vi "LSX Set Command Timeout.vi"(7 "lAtoCalibrate":i32, 8 "error in (no error)":errorcluster, 9 "lAtoMove":i32, 10 "lAtoRead":i32, 11 "lLSID":i32) -> (0 "error out":errorcluster, 3 "function return":i32)   [LabVIEW 2018, in "Tango.lvlib"]
doc: "TANGOAPI int TANGOCALL LSX_SetCommandTimeout (int lLSID, int lAtoRead, int lAtoMove, int lAtoCalibrate);"
uses:
  Tango.lvlib
  SubVIs/Tango_DLL.dll
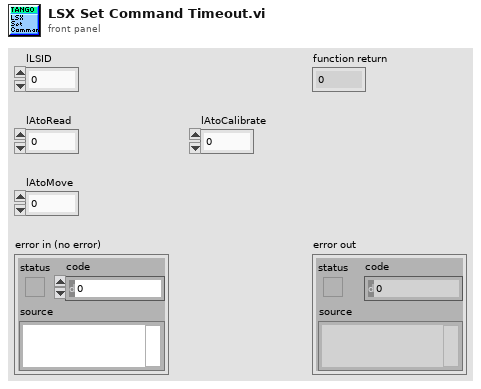
[diagram p1: front panel]
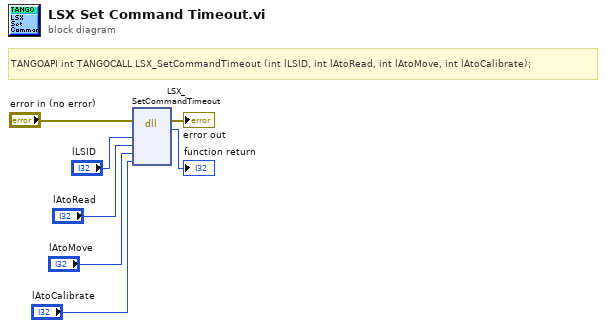
[diagram p0: block diagram]
diagram:
  # "TANGOAPI int TANGOCALL LSX_SetCommandTimeout (int lLSID, int lAtoRead, int lAtoMove, int lAtoCalibrate);"
  n1 = dll-call lib="C:/Users/Familie/Documents/LabviewIX81/lib/TANGO Stage/SubVIs/Tango_DLL.*" fn="LSX_SetCommandTimeout"(error in="error in (no error)", "lLSID"="lLSID", "lAtoRead"="lAtoRead", "lAtoMove"="lAtoMove", "lAtoCalibrate"="lAtoCalibrate") -> (error out=→"error out":errorcluster, →"function return":i32)  [unwired: 6 in, 1 out]
